vi "Load AFM Subpanel.vi"(0 "Ring in":refnum<vi>, 1 "Background Image":refnum<vi>, 3 "name or relative path":string, 5 "Inkscape File (.svg)":refnum<vi>, 7 "Lithography Data":T2(array[cluster]), 9 "Subpanel":refnum<vi>, 11 "error in (no error)":errorcluster, 12 "Run":refnum<vi>, 13 "base path":path, 14 "Abort":refnum<vi>) -> (6 "reference out":refnum<vi>, 15 "error out":errorcluster)   [LabVIEW 2019]
doc: "This VI opens an AFM subpanel."
uses:
  <userlib>/LevyLab/Relay Box/Typedefs/Resistor--enum.ctl
  <userlib>/LevyLab/Relay Box/Relay-Box.lvclass
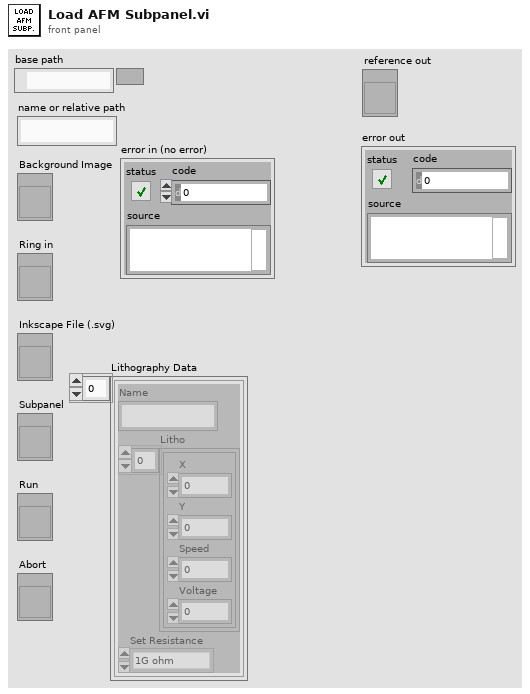
[diagram p1: front panel]
types:
  T1 = typedef "Relay-Box.lvclass/Resistor--enum.ctl" = enum16{"open", "discharge tip", "0 ohms", "100k ohm", "10M ohm", "1G ohm"}
  T2 = cluster{"Name":string, "Litho":cluster{"X":dbl, "Y":dbl, "Speed":dbl, "Voltage":dbl}[], "Set Resistance":T1}[]
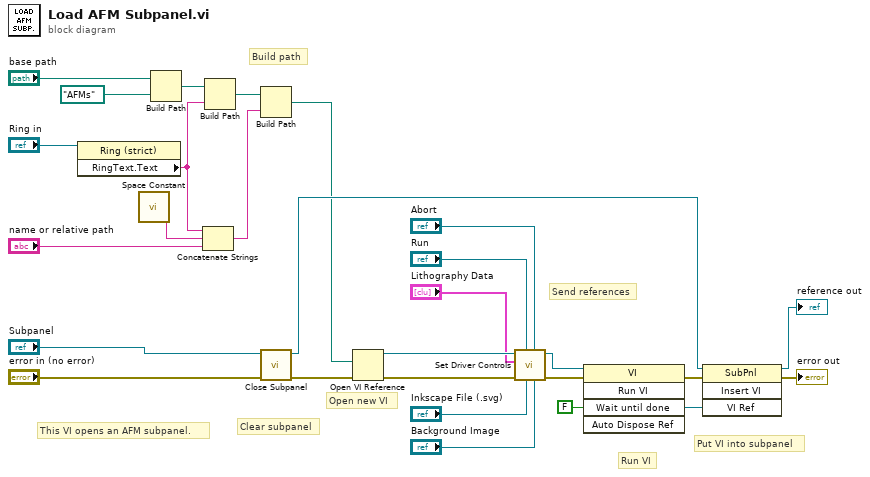
[diagram p0: block diagram]
diagram:
  # "This VI opens an AFM subpanel."
  # "Run VI"
  # "Put VI into subpanel"
  # "Send references"
  # "Open new VI"
  # "Clear subpanel"
  # "Build path"
  n1 = property class="Ring (strict)"(reference="Ring in") -> ("RingText.Text"=w2:string)  [unwired: 1 in, 2 out]
  n2 = call <vilib>:"Space Constant.vi"() -> ("String"=w3:string)
  n3 = Build Path(base path="base path", name or relative path=path "AFMs" ("path")) -> (appended path=w24:path)
  n4 = Concatenate Strings(w2, w3, "name or relative path") -> (w19:string)
  n5 = Build Path(base path=w24, name or relative path=w2) -> (appended path=w27:path)
  n6 = Build Path(base path=w27, name or relative path=w19) -> (appended path=w1:path)
  n7 = call "Close Subpanel.vi"("error in (no error)"="error in (no error)", "SubPanel in"="Subpanel") -> ("error out"=w28:errorcluster, "SubPanel out"=w5:refnum<vi>)  [unwired: 8 in]
  n8 = Open VI Reference(vi path=w1, error in (no error)=w28) -> (vi reference=w15:refnum<vi>, error out=w16:errorcluster)  [unwired: 4 in]
  n9 = call "Set Driver Controls.vi"("Background Image"="Background Image", "Abort"="Abort", "Inkscape File (.svg)"="Inkscape File (.svg)", "Run"="Run", "error in (no error)"=w16, "Lithography Data"="Lithography Data", "VI in"=w15) -> ("error out"=w17:errorcluster, "VI out"=w18:refnum<vi>)  [unwired: 3 in]
  n10 = invoke class="VI" method="Run VI"(reference=w18, error in=w17, "Wait until done"=FALSE ("Wait Until Done")) -> (reference out=w26:refnum<vi>, error out=w25:errorcluster)  [unwired: 2 in, 3 out]
  n11 = invoke class="SubPnl" method="Insert VI"(reference=w5, error in=w25, "VI Ref"=w26) -> (reference out=→"reference out":refnum<vi>, error out=→"error out":errorcluster)  [unwired: 1 in, 2 out]
